vi "PostCopyScripting.vi"(10 "MetaDataObj":refnum<class "MetaDataObj.lvclass">, 11 "User Project":refnum<vi>) -> ()   [LabVIEW 2019, in "MetaDataObj.Instrument.lvclass"]
uses:
  MetaDataObj.Instrument.lvclass
  <resource>/dialog/NewProjectWizard/MetaDataObj/MetaDataObj.lvclass
  <userlib>/_MGI/File/MGI Create Directory Chain Behavior Enum.ctl
panel:
  out "Status":string
  # "Creating Project..."
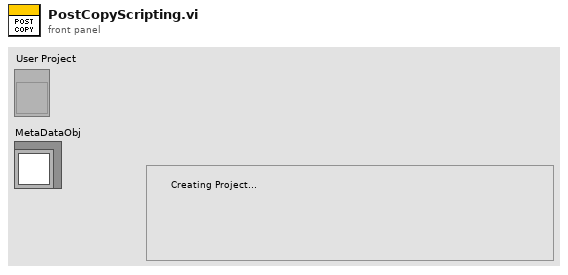
[diagram p1: front panel]
types:
  T1 = enum32{"Invalid", "Standard", "Closed", "Hidden", "Minimized", "Maximized"}
  T2 = enum32{"invalid app kind", "Development System", "Run Time System", "Student Edition", "Embedded LabVIEW", "Evaluation", "Custom"}
  T3 = typedef "MGI Create Directory Chain Behavior Enum.ctl" = enum16{"Auto Detect", "Path Contains a File", "Path Does Not Contain a File"}
  T4 = cluster{"Core":cluster{"Current VI Reference":refnum<vi>, "Close Panel on Exit?":bool}, "ProjectTemplate":path, "New Project Folder":path, "New Project File":path}
  T5 = cluster{"Current VI Reference":refnum<vi>, "Close Panel on Exit?":bool}
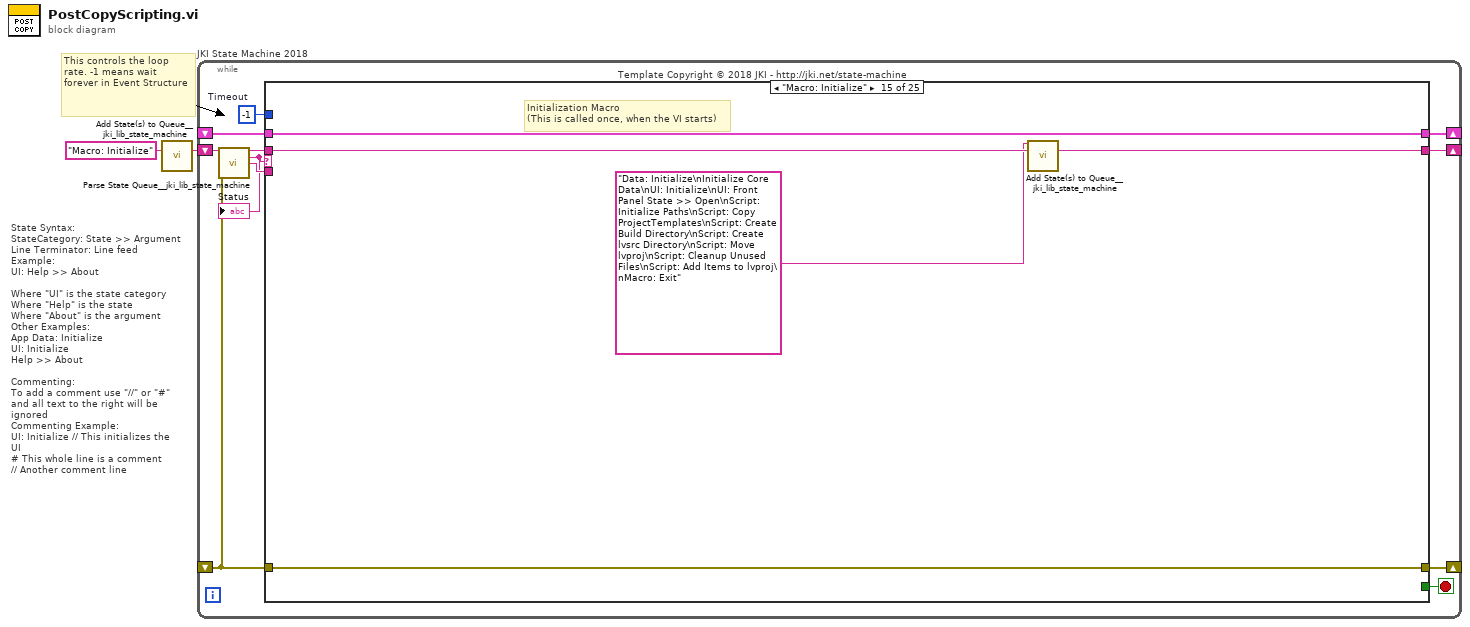
[diagram p0: block diagram]
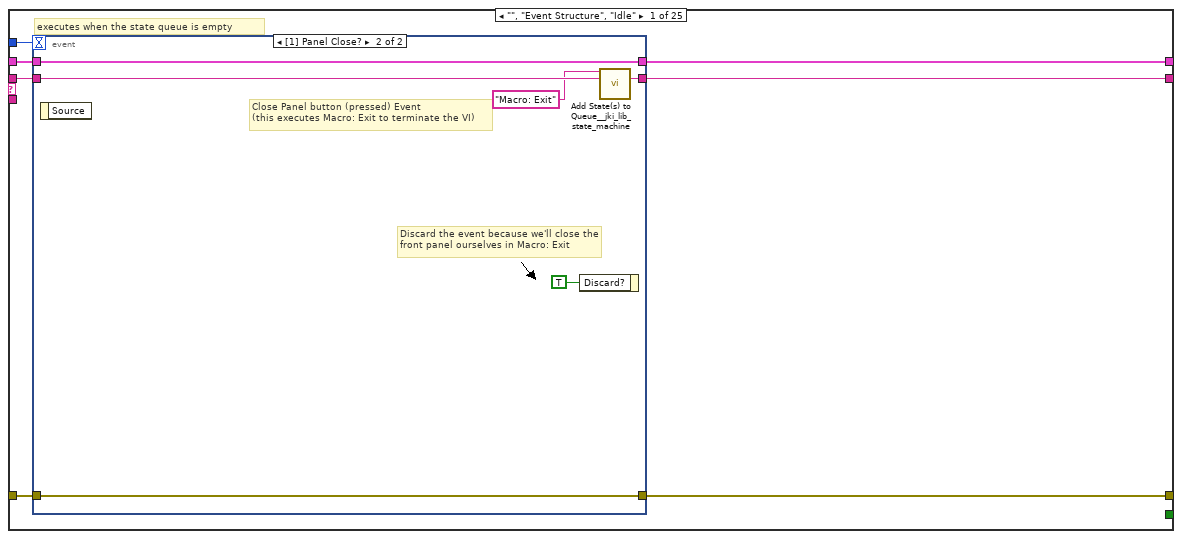
[diagram p2: hidden frame]
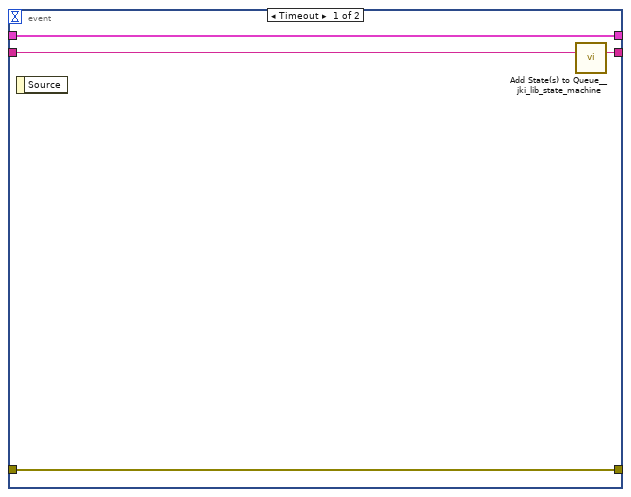
[diagram p3: hidden frame]
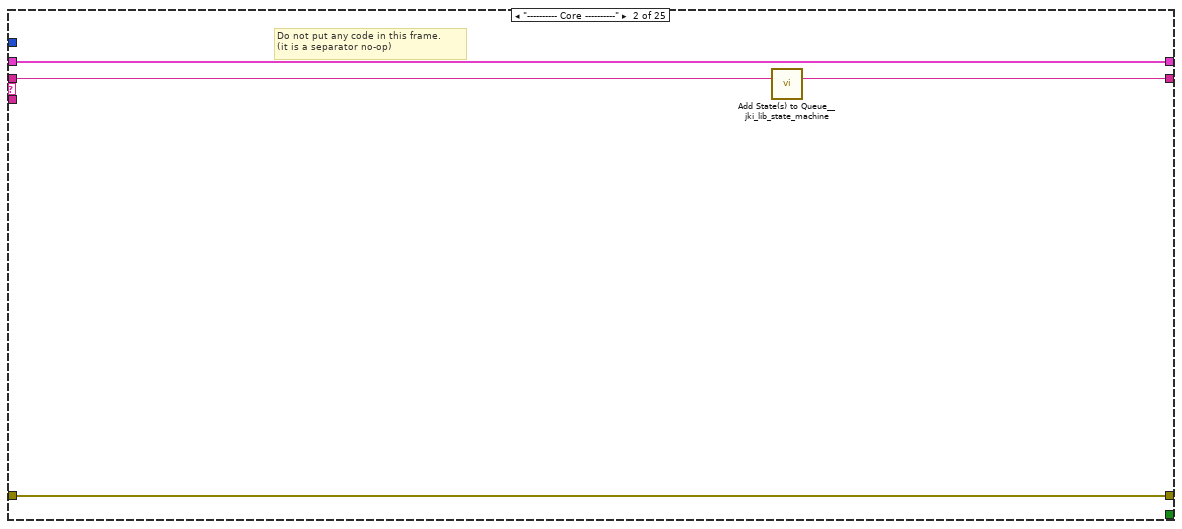
[diagram p4: hidden frame]
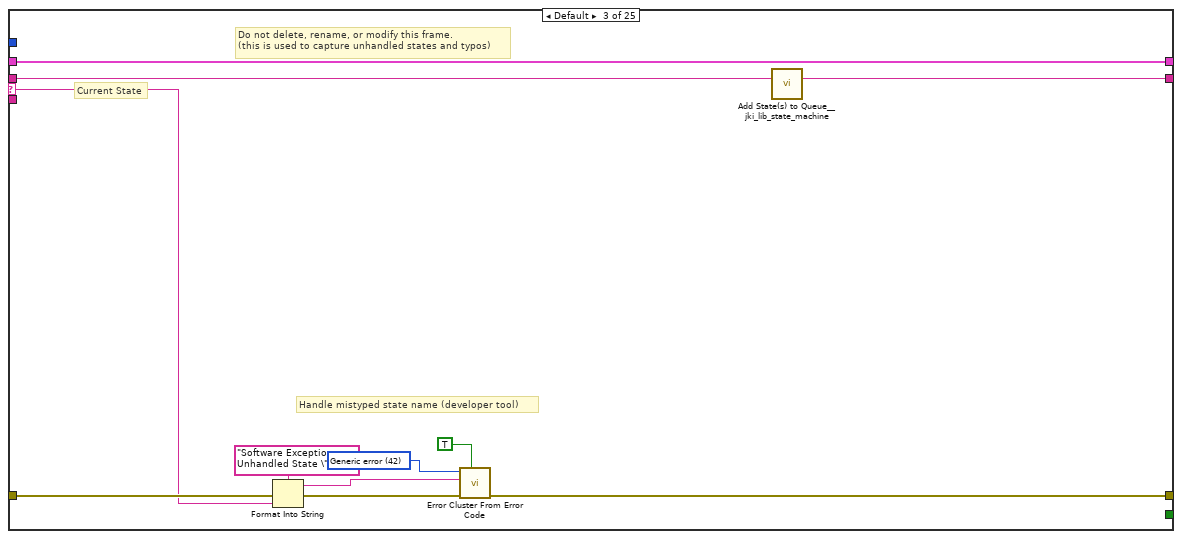
[diagram p5: hidden frame]
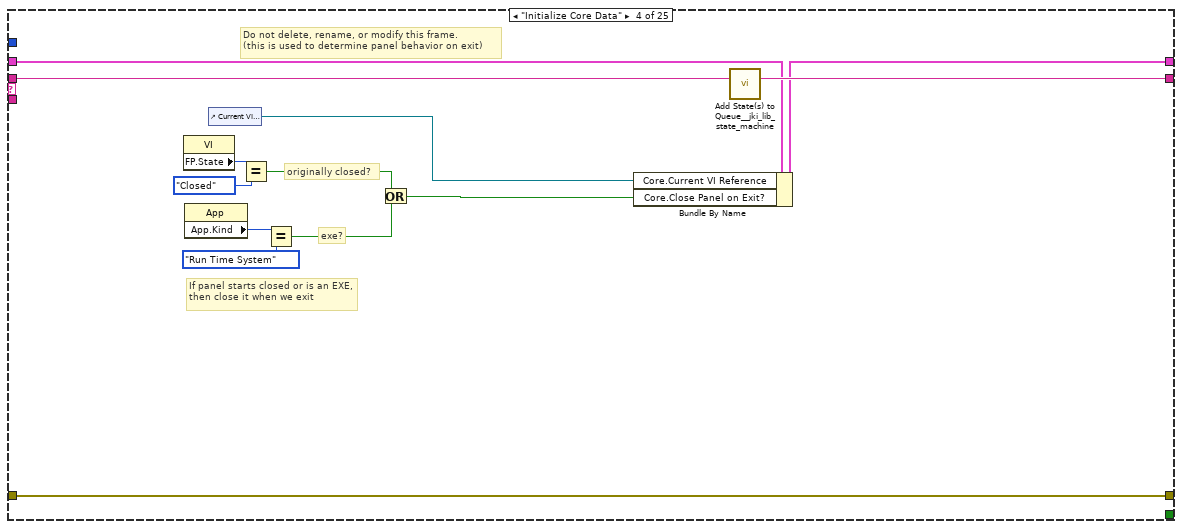
[diagram p6: hidden frame]
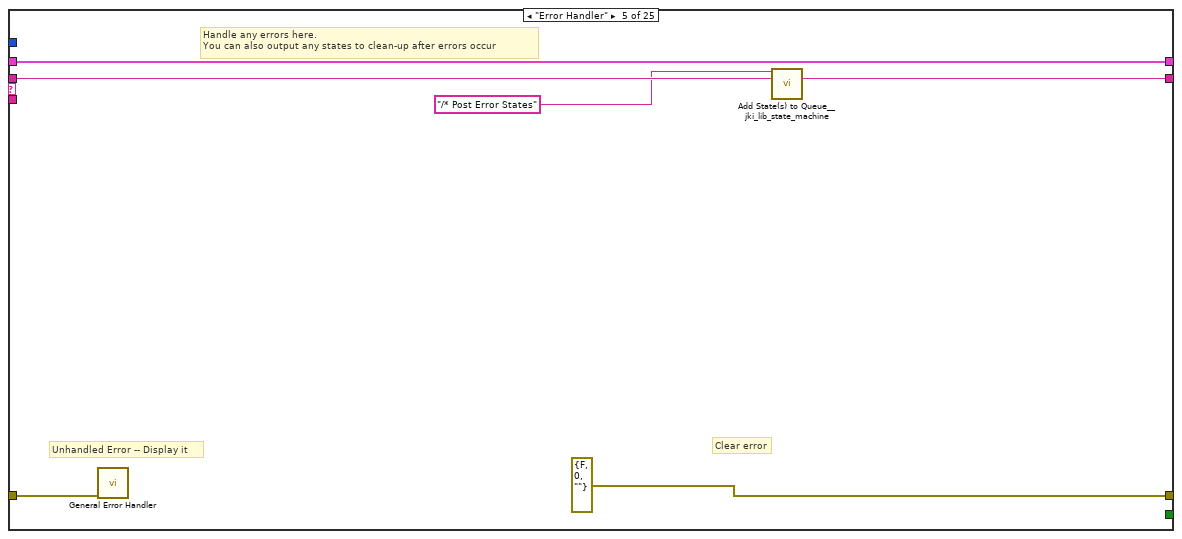
[diagram p7: hidden frame]
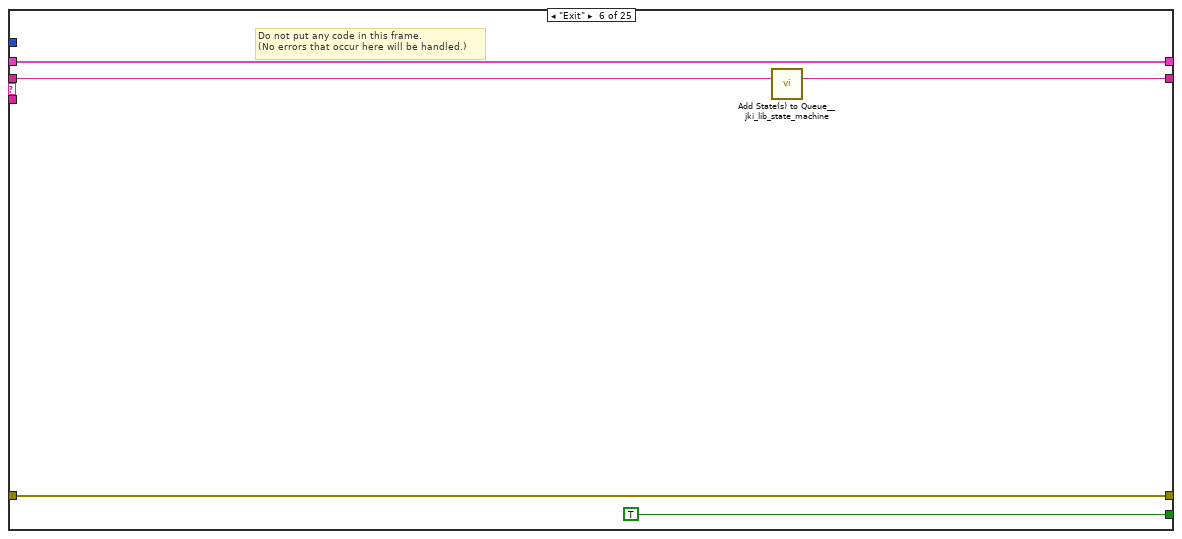
[diagram p8: hidden frame]
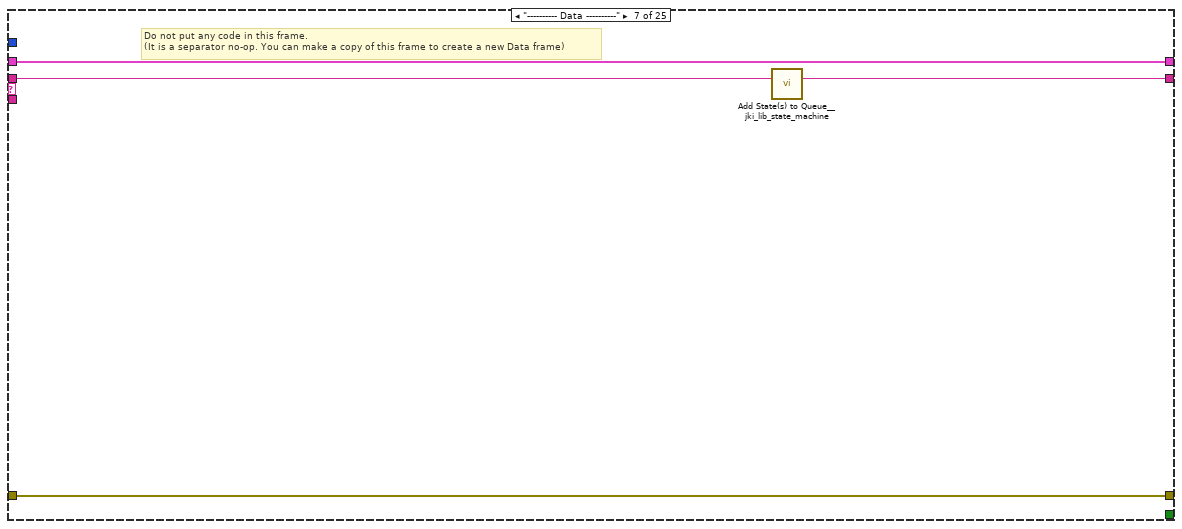
[diagram p9: hidden frame]
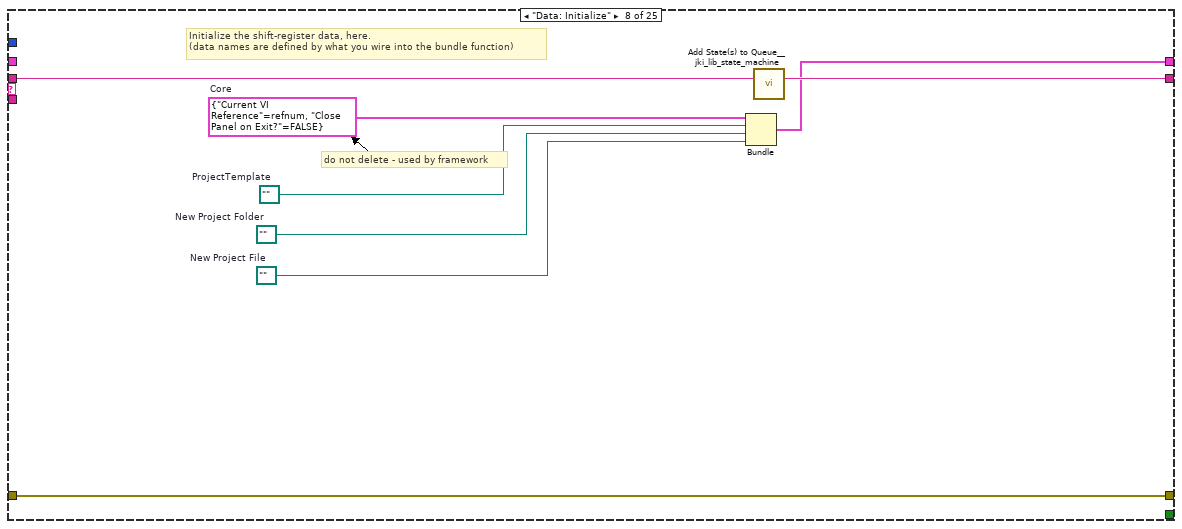
[diagram p10: hidden frame]
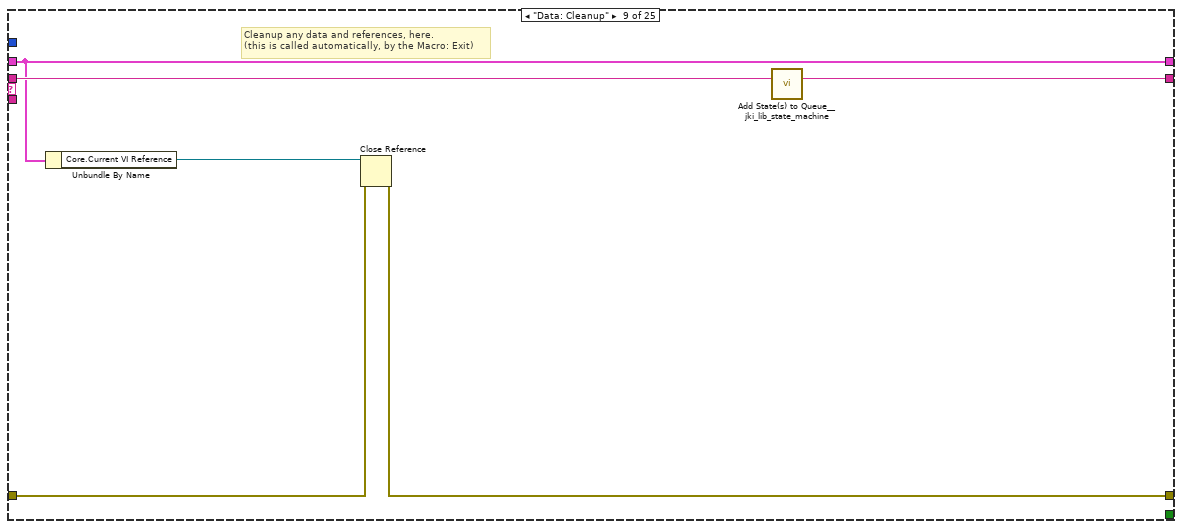
[diagram p11: hidden frame]
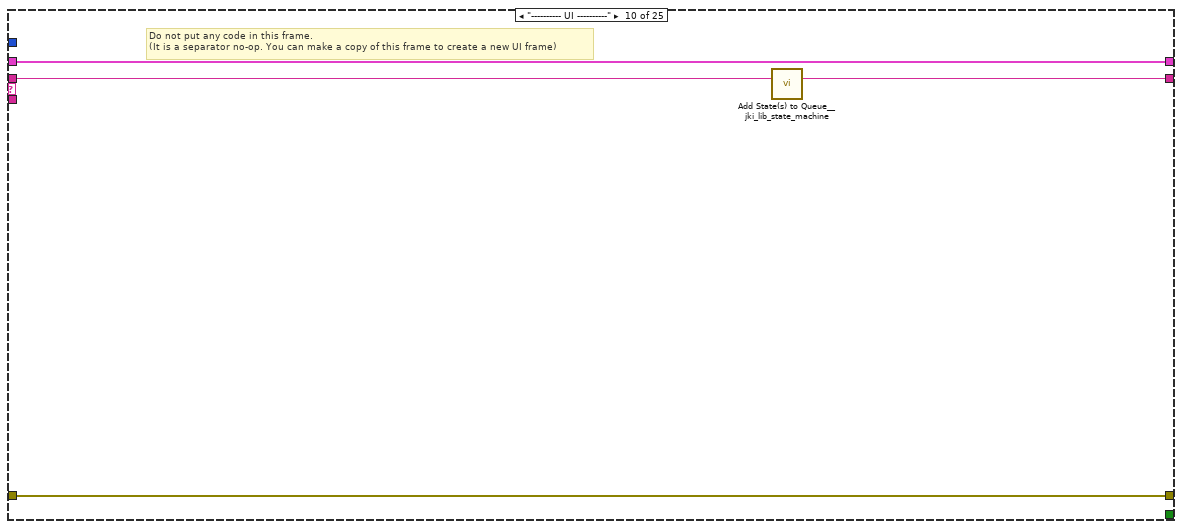
[diagram p12: hidden frame]
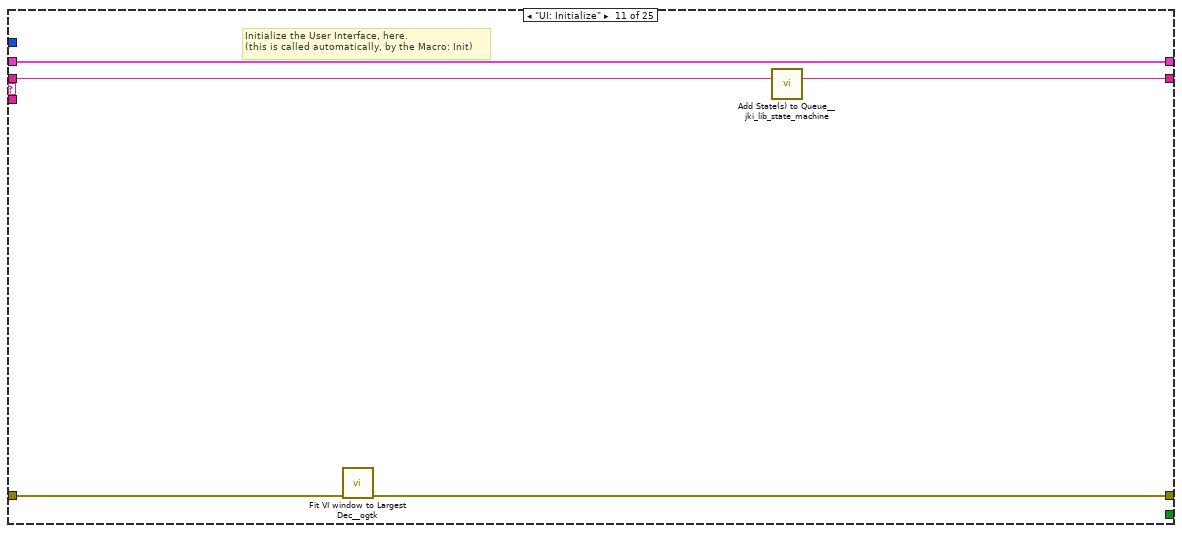
[diagram p13: hidden frame]
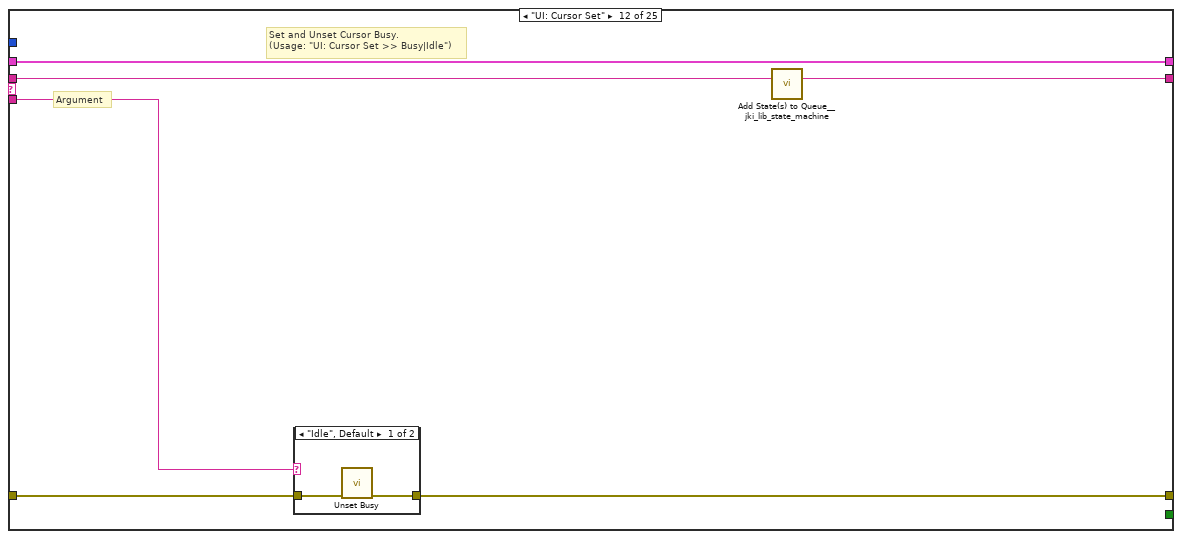
[diagram p14: hidden frame]
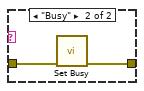
[diagram p15: hidden frame]
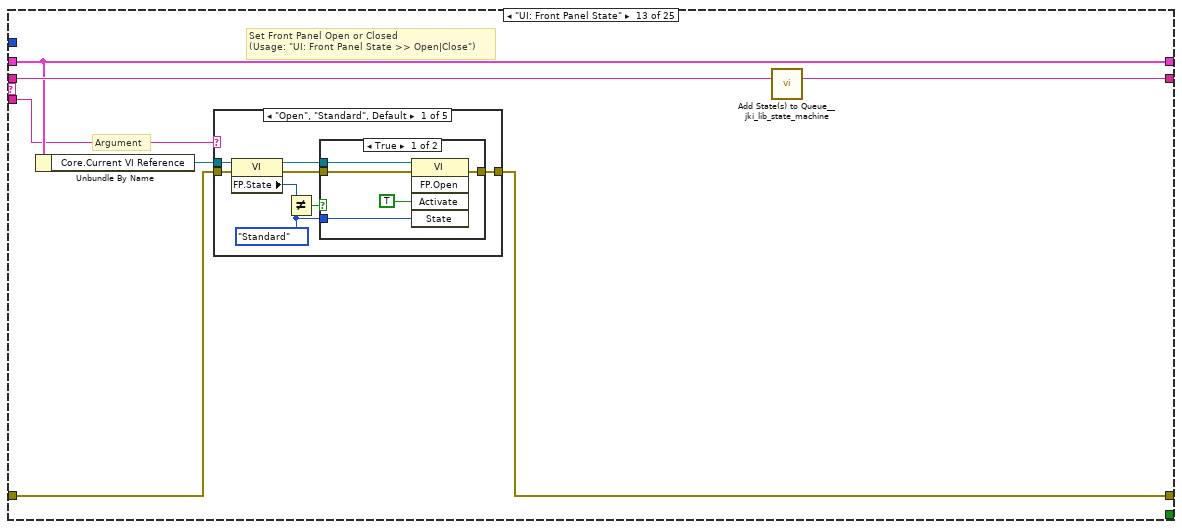
[diagram p16: hidden frame]
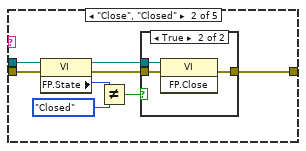
[diagram p18: hidden frame]
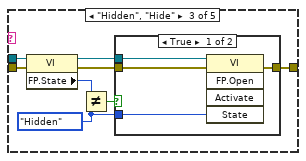
[diagram p20: hidden frame]
diagram:
  # "State Syntax:\nStateCategory: State >> Argument\nLine Terminator: Line feed\nExample:\nUI: Help >> About\n\nWhere \"UI\" is the state category\nWhere \"Help\" is the state\nWhere \"About\" is the argument\nOther Examples:\nApp Data: Initialize\nUI: Initialize\nHelp >> About\n\nCommenting:\nTo add a comment use \"//\" or \"#\" and all text to the right will be ignored\nCommenting Example:\nUI: Initialize // This initializes the UI\n# This whole line is a comment\n// Another comment line"
  # "This controls the loop rate. -1 means wait forever in Event Structure"
  n1 = call <vilib>:"Add State(s) to Queue__jki_lib_state_machine.vi"("State(s) in (\"\")"="Macro: Initialize") -> ("States Out"=w1:string)  [unwired: 14 in]
  n2 = while "JKI State Machine 2018" {
    shift-right: [w7] -> _
    shift-left: _ -> [w6]
    shift-right: [w10] -> _
    shift-left: _ -> [w4]
    shift-right: [w9] -> _
    shift-left: w1 -> [w11]
    stop <- w8 stop-if-true
    w5 = -1  # Timeout
    # "Template Copyright © 2018 JKI - http://jki.net/state-machine"
    n3 = call <vilib>:"Parse State Queue__jki_lib_state_machine.vi"("State Queue"=w11, "Error In (no error)"=w4) -> ("Remaining States"=w13:string, "Current State"=w3:string, "Arguments"=w12:string)  [unwired: 11 in]
    "Status" <- w3
    n4 = case shown="\"Macro: Initialize\"" w3 {
      selector: w3 -> [_ _ w35 _ _ _ _ _ _ _ _ _ _ _ _ _ _ _ _ _ _ _ _ _ _]
      tunnel: w13 -> [w20 w34 w39 w58 w64 w69 w73 w81 w87 w91 w96 w102 w113 w182 w187 w197 w201 w208 w223 w231 w269 w284 w300 w310 w338]
      tunnel: w12 -> [_ _ _ _ _ _ _ _ _ _ _ w97 w108 _ _ _ _ _ _ _ _ _ _ _ _]
      tunnel: w6 -> [w18 w31 w37 w51 w61 w67 w70 _ w82 w88 w94 w100 w110 w179 w184 w194 w198 w203 w217 w227 w263 w280 w287 w308 w336]
      tunnel: [w17 w32 w41 w55 errorcluster {"status"=FALSE, "code"=0, "source"=""} ("error out") w66 w71 w75 w83 w89 w92 w98 w107 w180 w185 w195 w199 w206 w221 w228 w261 w278 w289 w307 w320] -> w10
      tunnel: w4 -> [w16 w32 w40 w55 w60 w66 w71 w75 w84 w89 w93 w99 w111 w180 w185 w195 w199 w206 w221 w229 w262 w279 w290 w306 w335]
      tunnel: [w19 w33 w38 w57 w63 w68 w72 w80 w86 w90 w95 w101 w112 w181 w186 w196 w200 w207 w222 w230 w268 w283 w299 w309 w337] -> w9
      tunnel: [_ _ _ _ _ TRUE _ _ _ _ _ _ _ _ _ _ _ _ _ _ _ _ _ _ _] -> w8
      tunnel: [w15 w31 w37 w56 w61 w67 w70 w79 w82 w88 w94 w100 w110 w179 w184 w194 w198 w202 w216 w227 w263 w280 w286 w308 w336] -> w7
      tunnel: w5 -> [w14 _ _ _ _ _ _ _ _ _ _ _ _ _ _ _ _ _ _ _ _ _ _ _ _]
      frame "", "Event Structure", "Idle" {
        # "executes when the state queue is empty"
        n5 = event shown="[1] Panel Close?" {
          selector: _ -> [_ _]
          dyn-events: _ -> [_ _]
          timeout: w14 -> [_ _]
          tunnel: w20 -> [w24 w30]
          tunnel: [w23 w29] -> w19
          tunnel: w18 -> [w21 w27]
          tunnel: [w22 w28] -> w17
          tunnel: w16 -> [w22 w28]
          tunnel: [w21 w27] -> w15
          event Timeout {
            n6 = event-data() -> ()  [unwired: 1 in, 1 out]
            n7 = call <vilib>:"Add State(s) to Queue__jki_lib_state_machine.vi"("State(s) in (\"\")"=w24) -> ("States Out"=w23:string)  [unwired: 14 in]
          }
          event Panel Close? {
            # "Discard the event because we'll close the front panel ourselves in Macro: Exit"
            # "Close Panel button (pressed) Event\n(this executes Macro: Exit to terminate the VI)"
            n8 = event-data() -> ()  [unwired: 1 in, 1 out]
            n9 = event-data("Discard?"=TRUE) -> ()  [unwired: 1 in, 1 out]
            n10 = call <vilib>:"Add State(s) to Queue__jki_lib_state_machine.vi"("State(s) in Front (\"\")"="Macro: Exit", "State(s) in (\"\")"=w30) -> ("States Out"=w29:string)  [unwired: 13 in]
          }
        }
      }
      frame "---------- Core ----------" {
        # "Do not put any code in this frame.\n(it is a separator no-op)"
        n11 = call <vilib>:"Add State(s) to Queue__jki_lib_state_machine.vi"("State(s) in (\"\")"=w34) -> ("States Out"=w33:string)  [unwired: 14 in]
      }
      frame Default {
        w44 = 42 items=["No error", "Argument error", "Memory is full", "Out of zone", "End of file", "File already open", "Generic file I/O error", "File not found", "File permission error", "Disk is full", "Duplicate path", "Too many files open", "System feature not enabled", "Resource file not found", "Cannot add resource", "Resource not found", "Image not found", "Image memory error", "Pen does not exist", "Config type invalid", "Config token not found", "Config parse error", "Config memory error", "Bad external code format", "Bad external code offset", "External code not present", "Null window", "Destroy window error", "Null menu", "Print aborted", "Bad print record", "Print driver error", "Windows error during printing", "Memory error during printing", "Print dialog error", "Generic print error", "Invalid device refnum", "Device not found", "Device parameter error", "Device unit error", "Cannot open device", "Device call aborted", "Generic error", "Cancelled by user", "Object ID too low", "Object ID too high", "Object not in heap", "Unknown heap", "Unknown object (invalid DefProc)", "Unknown object (DefProc not in table)", "Message out of range", "Invalid (null) method", "Unknown message", "Manager call not supported", "Bad address", "Network operation in progress", "Network operation timed out", "Connection is busy", "Network attribute not supported", "Network error", "Address in use", "System out of memory", "Connection aborted", "Connection refused", "Not connected", "Already connected", "Connection closed", "Initialization error (interapplication manager)", "Bad occurrence", "Wait on unbound occurrence handler", "Occurrence queue overflow", "Datalog type conflict", "Unused", "Unrecognized type (interapplication manager)", "Memory corrupt", "Failed to make temporary DLL", "Old CIN version", "Drag socket not found", "Failed to load drop-object", "Failed to register OLE object", "Failed to release OLE object", "Format specifier type mismatch", "Unknown format specifier", "Too few format specifiers", "Too many format specifiers", "Scan failed", "Newer CIN version", "Error converting to variant", "Runtime menu error", "Password tampered", "Variant attribute not found", "Incompatible variant data type", "Event data is not available", "Event Store is not present", "Occurrence is not found", "Event Queue is not created", "Event info is not available", "Refnum passed is NULL", "Error retrieving Class GUID", "Error retrieving CoClass GUID", "Error retrieving TypeLib GUID.", "Bad built application magic bytes.", "Specific driver is different from the specific driver associated with the Logical Name.", "There is no session opened to the class driver.", "Max Error", "MAX - Error with config objects", "MAX - Error loading configuration", "MAX - Group not supported"]
        # "Current State"
        # "Do not delete, rename, or modify this frame.\n(this is used to capture unhandled states and typos)"
        # "Handle mistyped state name (developer tool)"
        n12 = Format Into String(format string="Software Exception: Unhandled State \"%s\"." ("message"), error in=w40, w35) -> (resulting string=w43:string, error out=w42:errorcluster)  [unwired: 1 in]
        n13 = call <vilib>:"Error Cluster From Error Code.vi"("show call chain? (False)"=TRUE, "error in (no error)"=w42, "error message (\"\")"=w43, "error code (0)"=w44) -> ("error out"=w41:errorcluster)  [unwired: 5 in]
        n14 = call <vilib>:"Add State(s) to Queue__jki_lib_state_machine.vi"("State(s) in (\"\")"=w39) -> ("States Out"=w38:string)  [unwired: 14 in]
      }
      frame "Initialize Core Data" {
        # "Do not delete, rename, or modify this frame.\n(this is used to determine panel behavior on exit)"
        # "originally closed?"
        # "exe?"
        # "If panel starts closed or is an EXE, then close it when we exit"
        n15 = property class="VI"() -> ("FP.State"=w48:T1)  [unwired: 2 in, 2 out]
        n16 = property class="App"() -> ("App.Kind"=w54:T2)  [unwired: 2 in, 2 out]
        n17 = control-ref of="Current VI Reference"() -> (w49:refnum<vi>)
        n18 = Equal?(x=w48, y=T1."Closed" ("Front Panel Window:State")) -> (x = y?=w46:bool)
        n19 = Equal?(x=w54, y=T2."Run Time System" ("Application:Kind")) -> (x = y?=w52:bool)
        n20 = Or(x=w46, y=w52) -> (x .or. y?=w50:bool)
        n21 = Bundle By Name(cluster=w51, "Core.Current VI Reference"=w49, "Core.Close Panel on Exit?"=w50) -> (w56:T4)
        n22 = call <vilib>:"Add State(s) to Queue__jki_lib_state_machine.vi"("State(s) in (\"\")"=w58) -> ("States Out"=w57:string)  [unwired: 14 in]
      }
      frame "Error Handler" {
        # "Unhandled Error -- Display it"
        # "Handle any errors here.\nYou can also output any states to clean-up after errors occur"
        # "Clear error"
        n23 = call <vilib>:"General Error Handler.vi"("error in (no error)"=w60) -> ()  [unwired: 10 in, 5 out]
        n24 = call <vilib>:"Add State(s) to Queue__jki_lib_state_machine.vi"("State(s) in Front (\"\")"="/* Post Error States", "State(s) in (\"\")"=w64) -> ("States Out"=w63:string)  [unwired: 13 in]
      }
      frame "Exit" {
        # "Do not put any code in this frame.\n(No errors that occur here will be handled.)"
        n25 = call <vilib>:"Add State(s) to Queue__jki_lib_state_machine.vi"("State(s) in (\"\")"=w69) -> ("States Out"=w68:string)  [unwired: 14 in]
      }
      frame "---------- Data ----------" {
        # "Do not put any code in this frame.\n(It is a separator no-op. You can make a copy of this frame to create a new Data frame)"
        n26 = call <vilib>:"Add State(s) to Queue__jki_lib_state_machine.vi"("State(s) in (\"\")"=w73) -> ("States Out"=w72:string)  [unwired: 14 in]
      }
      frame "Data: Initialize" {
        w74 = path ""  # New Project File
        w76 = path ""  # ProjectTemplate
        w77 = path ""  # New Project Folder
        w78 = T5 {"Current VI Reference"=refnum, "Close Panel on Exit?"=FALSE}  # Core
        # "do not delete - used by framework"
        # "Initialize the shift-register data, here.\n(data names are defined by what you wire into the bundle function)"
        n27 = Bundle("Core"=w78, "ProjectTemplate"=w76, "New Project Folder"=w77, "New Project File"=w74) -> (w79:T4)  [unwired: 1 in]
        n28 = call <vilib>:"Add State(s) to Queue__jki_lib_state_machine.vi"("State(s) in (\"\")"=w81) -> ("States Out"=w80:string)  [unwired: 14 in]
      }
      frame "Data: Cleanup" {
        # "Cleanup any data and references, here.\n(this is called automatically, by the Macro: Exit)"
        n29 = Unbundle By Name(w82) -> ("Core.Current VI Reference"=w85:refnum<vi>)
        n30 = Close Reference(reference=w85, error in (no error)=w84) -> (error out=w83:errorcluster)
        n31 = call <vilib>:"Add State(s) to Queue__jki_lib_state_machine.vi"("State(s) in (\"\")"=w87) -> ("States Out"=w86:string)  [unwired: 14 in]
      }
      frame "---------- UI ----------" {
        # "Do not put any code in this frame.\n(It is a separator no-op. You can make a copy of this frame to create a new UI frame)"
        n32 = call <vilib>:"Add State(s) to Queue__jki_lib_state_machine.vi"("State(s) in (\"\")"=w91) -> ("States Out"=w90:string)  [unwired: 14 in]
      }
      frame "UI: Initialize" {
        # "Initialize the User Interface, here.\n(this is called automatically, by the Macro: Init)"
        n33 = call <userlib>:"Fit VI window to Largest Dec__ogtk.vi"("error in (no error)"=w93) -> ("error out"=w92:errorcluster)  [unwired: 5 in, 1 out]
        n34 = call <vilib>:"Add State(s) to Queue__jki_lib_state_machine.vi"("State(s) in (\"\")"=w96) -> ("States Out"=w95:string)  [unwired: 14 in]
      }
      frame "UI: Cursor Set" {
        # "Argument"
        # "Set and Unset Cursor Busy.\n(Usage: \"UI: Cursor Set >> Busy|Idle\")"
        n35 = case shown="\"Idle\", Default" w97 {
          tunnel: w99 -> [w104 w106]
          tunnel: [w103 w105] -> w98
          frame "Idle", Default {
            n36 = call <vilib>:"Unset Busy.vi"("error in (no error)"=w104) -> ("error out"=w103:errorcluster)  [unwired: 10 in]
          }
          frame "Busy" {
            n37 = call <vilib>:"Set Busy.vi"("error in (no error)"=w106) -> ("error out"=w105:errorcluster)  [unwired: 9 in, 1 out]
          }
        }
        n38 = call <vilib>:"Add State(s) to Queue__jki_lib_state_machine.vi"("State(s) in (\"\")"=w102) -> ("States Out"=w101:string)  [unwired: 14 in]
      }
      frame "UI: Front Panel State" {
        # "Argument"
        # "Set Front Panel Open or Closed\n(Usage: \"UI: Front Panel State >> Open|Close\")"
        n39 = Unbundle By Name(w110) -> ("Core.Current VI Reference"=w109:refnum<vi>)
        n40 = case shown="\"Open\", \"Standard\", Default" w108 {
          tunnel: w111 -> [w119 w134 w145 w158 w171]
          tunnel: [w121 w135 w147 w160 w173] -> w107
          tunnel: w109 -> [w120 w132 w146 w159 w172]
          frame "Open", "Standard", Default {
            w114 = T1."Standard" ("State")
            n41 = property class="VI"(reference=w120, error in=w119) -> (reference out=w117:refnum<vi>, error out=w118:errorcluster, "FP.State"=w116:T1)
            n42 = Not Equal?(x=w116, y=w114) -> (x != y?=w115:bool)
            n43 = case shown="True" w115 {
              tunnel: [w125 w127] -> w121
              tunnel: w118 -> [w124 w127]
              tunnel: w117 -> [w123 _]
              tunnel: w114 -> [w122 _]
              frame True {
                n44 = invoke class="VI" method="FP.Open"(reference=w123, error in=w124, "Activate"=TRUE, "State"=w122) -> (error out=w125:errorcluster)  [unwired: 1 in, 4 out]
              }
              frame False {
              }
            }
          }
          frame "Close", "Closed" {
            n45 = property class="VI"(reference=w132, error in=w134) -> (reference out=w131:refnum<vi>, error out=w133:errorcluster, "FP.State"=w129:T1)
            n46 = Not Equal?(x=w129, y=T1."Closed" ("Front Panel Window:State")) -> (x != y?=w128:bool)
            n47 = case shown="True" w128 {
              tunnel: [w136 w139] -> w135
              tunnel: w133 -> [w136 w138]
              tunnel: w131 -> [_ w137]
              frame False {
              }
              frame True {
                n48 = invoke class="VI" method="FP.Close"(reference=w137, error in=w138) -> (error out=w139:errorcluster)  [unwired: 1 in, 2 out]
              }
            }
          }
          frame "Hidden", "Hide" {
            w140 = T1."Hidden" ("State")
            n49 = property class="VI"(reference=w146, error in=w145) -> (reference out=w143:refnum<vi>, error out=w144:errorcluster, "FP.State"=w142:T1)
            n50 = Not Equal?(x=w142, y=w140) -> (x != y?=w141:bool)
            n51 = case shown="True" w141 {
              tunnel: [w151 w152] -> w147
              tunnel: w144 -> [w150 w152]
              tunnel: w143 -> [w149 _]
              tunnel: w140 -> [w148 _]
              frame True {
                n52 = invoke class="VI" method="FP.Open"(reference=w149, error in=w150, "State"=w148) -> (error out=w151:errorcluster)  [unwired: 2 in, 4 out]
              }
              frame False {
              }
            }
          }
          frame "Minimize", "Minimized" {
            w153 = T1."Minimized" ("State")
            n53 = property class="VI"(reference=w159, error in=w158) -> (reference out=w156:refnum<vi>, error out=w157:errorcluster, "FP.State"=w155:T1)
            n54 = Not Equal?(x=w155, y=w153) -> (x != y?=w154:bool)
            n55 = case shown="True" w154 {
              tunnel: [w164 w165] -> w160
              tunnel: w157 -> [w163 w165]
              tunnel: w156 -> [w162 _]
              tunnel: w153 -> [w161 _]
              frame True {
                n56 = invoke class="VI" method="FP.Open"(reference=w162, error in=w163, "State"=w161) -> (error out=w164:errorcluster)  [unwired: 2 in, 4 out]
              }
              frame False {
              }
            }
          }
          frame "Maximize", "Maximized" {
            w166 = T1."Maximized" ("State")
            n57 = property class="VI"(reference=w172, error in=w171) -> (reference out=w169:refnum<vi>, error out=w170:errorcluster, "FP.State"=w168:T1)
            n58 = Not Equal?(x=w168, y=w166) -> (x != y?=w167:bool)
            n59 = case shown="True" w167 {
              tunnel: [w177 w178] -> w173
              tunnel: w170 -> [w176 w178]
              tunnel: w169 -> [w175 _]
              tunnel: w166 -> [w174 _]
              frame True {
                n60 = invoke class="VI" method="FP.Open"(reference=w175, error in=w176, "State"=w174) -> (error out=w177:errorcluster)  [unwired: 2 in, 4 out]
              }
              frame False {
              }
            }
          }
        }
        n61 = call <vilib>:"Add State(s) to Queue__jki_lib_state_machine.vi"("State(s) in (\"\")"=w113) -> ("States Out"=w112:string)  [unwired: 14 in]
      }
      frame "---------- Macro ----------" {
        # "Do not put any code in this frame.\n(It is a separator no-op. You can make a copy of this frame to create a new Macro frame)"
        n62 = call <vilib>:"Add State(s) to Queue__jki_lib_state_machine.vi"("State(s) in (\"\")"=w182) -> ("States Out"=w181:string)  [unwired: 14 in]
      }
      frame "Macro: Initialize" {
        # "Initialization Macro\n(This is called once, when the VI starts)"
        n63 = call <vilib>:"Add State(s) to Queue__jki_lib_state_machine.vi"("State(s) in Front (\"\")"="Data: Initialize\nInitialize Core Data\nUI: Initialize\nUI: Front Panel State >> Open\nScript: Initialize Paths\nScript: Copy ProjectTemplates\nScript: Create Build Directory\nScript: Create lvsrc Directory\nScript: Move lvproj\nScript: Cleanup Unused Files\nScript: Add Items to lvproj\nMacro: Exit", "State(s) in (\"\")"=w187) -> ("States Out"=w186:string)  [unwired: 13 in]
      }
      frame "Macro: Exit" {
        # "Exit Macro\n(This is called once, when the VI exits)"
        n64 = Unbundle By Name(w194) -> ("Core.Close Panel on Exit?"=w193:bool)
        n65 = Select(t="UI: Front Panel State >> Close", s=w193, f="") -> (s? t:f=w190:string)
        n66 = call <vilib>:"Add State(s) to Queue__jki_lib_state_machine.vi"("State(s) in (\"\")"=w190, "State(s) at Back (\"\")"="Data: Cleanup\nExit") -> ("States Out"=w188:string)  [unwired: 13 in]
        n67 = call <vilib>:"Add State(s) to Queue__jki_lib_state_machine.vi"("State(s) in Front (\"\")"=w188, "State(s) in (\"\")"=w197) -> ("States Out"=w196:string)  [unwired: 13 in]
      }
      frame "---------- Script ----------" {
        # "Template Separator\n(You can make a copy of, or modify, this frame)"
        n68 = call <vilib>:"Add State(s) to Queue__jki_lib_state_machine.vi"("State(s) in (\"\")"=w201) -> ("States Out"=w200:string)  [unwired: 14 in]
      }
      frame "Script: Template" {
        # "Your code here.\n(You can make a copy of, or modify, this frame)"
        n69 = Unbundle By Name(w203) -> ("ProjectTemplate"=w205:path, "New Project Folder"=w204:path)
        n70 = Bundle By Name(cluster=w203, "ProjectTemplate"=w205, "New Project Folder"=w204) -> (w202:T4)
        n71 = call <vilib>:"Add State(s) to Queue__jki_lib_state_machine.vi"("State(s) in (\"\")"=w208) -> ("States Out"=w207:string)  [unwired: 14 in]
      }
      frame "Script: Initialize Paths" {
        w210 = refnum<class "MetaDataObj.Instrument.lvclass"> refnum  # MetaDataObj.Instrument.lvclass
        # "path to new project source"
        # "path to ProjectTemplate location"
        # "LabVIEW directory"
        # "Initialize Paths.\n(description)"
        n72 = property class="Project"(reference="User Project") -> (reference out=w214:refnum<vi>, error out=w213:errorcluster, "Path"=w209:path)  [unwired: 1 in]
        n73 = Default Directory() -> (w220:path)
        n74 = To More Specific Class(target class=w210, reference="MetaDataObj") -> ()  [unwired: 1 in, 2 out]
        n75 = Build Path(base path=w220, name or relative path="ProjectTemplates\\Source\\LevyLab\\Instrument\\project files") -> (appended path=w218:path)
        n76 = Close Reference(reference=w214, error in (no error)=w213) -> ()  [unwired: 1 out]
        n77 = Strip Path(path=w209) -> (stripped path=w215:path)  [unwired: 1 out]
        n78 = Bundle By Name(cluster=w217, "ProjectTemplate"=w218, "New Project Folder"=w215) -> (w216:T4)
        n79 = call <vilib>:"Add State(s) to Queue__jki_lib_state_machine.vi"("State(s) in (\"\")"=w223) -> ("States Out"=w222:string)  [unwired: 14 in]
      }
      frame "Script: Copy ProjectTemplates" {
        # "Copy code from ProjectTemplate to Source.\n(copy fiels that the Create Project dialog won't copy)"
        n80 = Unbundle By Name(w227) -> ("ProjectTemplate"=w225:path, "New Project Folder"=w226:path)
        n81 = for {
          tunnel: w226 -> [w242]
          shift-right: [w235] -> w228
          shift-left: w229 -> [w238]
          tunnel: string[] ["", "build support"] -> [w232] mode=indexing
          tunnel: w225 -> [w234]
          n82 = case shown="Default" w232 {
            selector: w232 -> [_ w246]
            tunnel: w234 -> [w245 w248]
            tunnel: [w245 w247] -> w233
            frame "" {
            }
            frame Default {
              n83 = Build Path(base path=w248, name or relative path=w246) -> (appended path=w247:path)
            }
          }
          n84 = case shown="Default" w232 {
            selector: w232 -> [_ w250]
            tunnel: w242 -> [w249 w252]
            tunnel: [w249 w251] -> w241
            frame "" {
            }
            frame Default {
              n85 = Build Path(base path=w252, name or relative path=w250) -> (appended path=w251:path)
            }
          }
          n86 = List Folder(path=w233, error in=w238) -> (path out=w244:path, filenames=w243:string[], error out=w237:errorcluster)  [unwired: 2 in, 1 out]
          n87 = call <userlib>:"MGI Create Directory Chain.vi"("Error In"=w237, "File Presence (Auto Detect)"=MGI_Create_Directory_Chain_Behavior_Enum."Auto Detect", "Path"=w241) -> ("Error Out"=w236:errorcluster, "Duplicate Path"=w240:path)  [unwired: 7 in]
          n88 = for {
            tunnel: w244 -> [w260]
            tunnel: w243 -> [w258] mode=indexing
            tunnel: w240 -> [w259]
            shift-right: [w253] -> w235
            shift-left: w236 -> [w256]
            n89 = Build Path(base path=w260, name or relative path=w258) -> (appended path=w254:path)
            n90 = Build Path(base path=w259, name or relative path=w258) -> (appended path=w255:path)
            n91 = Copy(8:w256, 9:TRUE ("overwrite (F)"), 10:w255, 11:w254) -> (0:w253:errorcluster)  [unwired: 1 in, 2 out]
          }
        }
        n92 = call <vilib>:"Add State(s) to Queue__jki_lib_state_machine.vi"("State(s) in (\"\")"=w231) -> ("States Out"=w230:string)  [unwired: 14 in]
      }
      frame "Script: Create Build Directory" {
        # "Create default builds/subfolder structure."
        n93 = Unbundle By Name(w263) -> ("New Project Folder"=w266:path)
        n94 = Build Path(base path=w266, name or relative path="builds") -> (appended path=w264:path)
        n95 = for {
          shift-right: [w270] -> w261
          shift-left: w262 -> [w274]
          tunnel: w264 -> [w273]
          tunnel: string[] ["7z Install", "Application", "Installer", "Latest", "Package"] -> [w272] mode=indexing
          tunnel: [w270] -> _ mode=indexing
          n96 = Build Path(base path=w273, name or relative path=w272) -> (appended path=w271:path)
          n97 = call <userlib>:"MGI Create Directory Chain.vi"("Error In"=w274, "File Presence (Auto Detect)"=MGI_Create_Directory_Chain_Behavior_Enum."Auto Detect", "Path"=w271) -> ("Error Out"=w270:errorcluster)  [unwired: 7 in, 1 out]
        }
        n98 = call <vilib>:"Add State(s) to Queue__jki_lib_state_machine.vi"("State(s) in (\"\")"=w269) -> ("States Out"=w268:string)  [unwired: 14 in]
      }
      frame "Script: Create lvsrc Directory" {
        # "Create lvsrc/ folder."
        n99 = Unbundle By Name(w280) -> ("New Project Folder"=w282:path)
        n100 = Build Path(base path=w282, name or relative path="lvsrc\\SMOs") -> (appended path=w276:path)
        n101 = call <userlib>:"MGI Create Directory Chain.vi"("Error In"=w279, "File Presence (Auto Detect)"=MGI_Create_Directory_Chain_Behavior_Enum."Auto Detect", "Path"=w276) -> ("Error Out"=w278:errorcluster)  [unwired: 7 in, 1 out]
        n102 = call <vilib>:"Add State(s) to Queue__jki_lib_state_machine.vi"("State(s) in (\"\")"=w284) -> ("States Out"=w283:string)  [unwired: 14 in]
      }
      frame "Script: Move lvproj" {
        # "Move *.lvproj from root to lvsrc/"
        n103 = Unbundle By Name(w287) -> ("New Project Folder"=w291:path)
        n104 = call <vilib>:"Recursive File List.vi"("pattern"="*.lvproj", "error in (no error)"=w290, "Folder Path"=w291) -> ("error out"=w294:errorcluster, "All Files in Dir"=w285:path[])  [unwired: 4 in, 3 out]
        n105 = Build Path(base path=w291, name or relative path="lvsrc") -> (appended path=w297:path)
        n106 = Index Array(array=w285) -> (element=w296:path)  [unwired: 1 in]
        n107 = Strip Path(path=w296) -> (name=w292:string)  [unwired: 1 out]
        n108 = Build Path(base path=w297, name or relative path=w292) -> (appended path=w298:path)
        n109 = Move(source path=w296, error in=w294, 10:w298) -> (error out=w289:errorcluster, 3:w288:path)  [unwired: 2 in, 1 out]
        n110 = Bundle By Name(cluster=w287, "New Project File"=w288) -> (w286:T4)
        n111 = call <vilib>:"Add State(s) to Queue__jki_lib_state_machine.vi"("State(s) in (\"\")"=w300) -> ("States Out"=w299:string)  [unwired: 14 in]
      }
      frame "Script: Cleanup Unused Files" {
        # "Delete uneeded files."
        n112 = Unbundle By Name(w308) -> ("New Project Folder"=w305:path)
        n113 = Build Array("*.aliases" ("pattern"), "*.lvlps" ("pattern"), "*.rename" ("pattern")) -> (w301:string[])
        n114 = for {
          tunnel: w305 -> [w312]
          shift-right: [w316] -> w307
          shift-left: w306 -> [w313]
          tunnel: w301 -> [w311] mode=indexing
          n115 = call <vilib>:"Recursive File List.vi"("pattern"=w311, "error in (no error)"=w313, "Folder Path"=w312) -> ("error out"=w315:errorcluster, "All Files in Dir"=w314:path[])  [unwired: 4 in, 3 out]
          n116 = for {
            tunnel: w314 -> [w319] mode=indexing
            shift-right: [w317] -> w316
            shift-left: w315 -> [w318]
            n117 = Delete(path (use dialog)=w319, error in=w318) -> (error out=w317:errorcluster)  [unwired: 3 in, 2 out]
          }
        }
        n118 = call <vilib>:"Add State(s) to Queue__jki_lib_state_machine.vi"("State(s) in (\"\")"=w310) -> ("States Out"=w309:string)  [unwired: 14 in]
      }
      frame "Script: Add Items to lvproj" {
        # "Add items to the Project"
        n119 = Unbundle By Name(w336) -> ("New Project Folder"=w332:path, "New Project File"=w330:path)
        n120 = invoke class="App" method="Project.Open"(error in=w335, "Path"=w330) -> (error out=w328:errorcluster, "Project:Open"=w329:refnum<vi>)  [unwired: 2 in, 2 out]
        n121 = invoke class="Project" method="Open Window"(reference=w329, error in=w328) -> (reference out=w327:refnum<vi>, error out=w326:errorcluster)  [unwired: 1 in, 1 out]
        n122 = property class="Project"(reference=w327, error in=w326) -> (reference out=w323:refnum<vi>, error out=w334:errorcluster, "My Computer"=w333:refnum<vi>)
        n123 = for "Add Folders" {
          tunnel: w334 -> [w349]
          tunnel: w333 -> [w347]
          tunnel: string[] ["build support", "lvsrc"] -> [w342] mode=indexing
          tunnel: w332 -> [w340]
          tunnel: [w344] -> w331
          n124 = Build Path(base path=w340, name or relative path=w342) -> (appended path=w339:path)
          n125 = invoke class="TargetItem" method="AddItem"(reference=w347, error in=w349, "Name"=w342, "Path"=w339, "Type"="Folder") -> (error out=w346:errorcluster, "AddItem"=w343:refnum<vi>)  [unwired: 1 in, 4 out]
          n126 = case shown="Default" w342 {
            tunnel: w346 -> [w351 w356]
            tunnel: [w351 w355] -> w345
            tunnel: w339 -> [_ w354]
            tunnel: w343 -> [w350 w353]
            tunnel: [w350 w352] -> w341
            frame "lvsrc" {
            }
            frame Default {
              n127 = call <vilib>:"Recursive File List.vi"("error in (no error)"=w356, "Folder Path"=w354) -> ("error out"=w358:errorcluster, "All Files in Dir"=w357:path[])  [unwired: 5 in, 3 out]
              n128 = for "Add Folder Contents" {
                tunnel: w353 -> [w360]
                tunnel: w357 -> [w363] mode=indexing
                tunnel: w358 -> [w365]
                tunnel: [w362] -> w355
                tunnel: [w359] -> w352
                n129 = invoke class="ProjectItem" method="AddFile"(reference=w360, error in=w365, "Path"=w363) -> (reference out=w359:refnum<vi>, error out=w364:errorcluster, "AddFile"=w361:refnum<vi>)  [unwired: 1 in, 1 out]
                n130 = Close Reference(reference=w361, error in (no error)=w364) -> (error out=w362:errorcluster)
              }
            }
          }
          n131 = Close Reference(reference=w341, error in (no error)=w345) -> (error out=w344:errorcluster)
        }
        n132 = Close Reference(reference=w333, error in (no error)=w331) -> (error out=w324:errorcluster)
        n133 = invoke class="Project" method="Save"(reference=w323, error in=w324) -> (reference out=w322:refnum<vi>, error out=w321:errorcluster)  [unwired: 2 in, 2 out]
        n134 = Close Reference(reference=w322, error in (no error)=w321) -> (error out=w320:errorcluster)
        n135 = call <vilib>:"Add State(s) to Queue__jki_lib_state_machine.vi"("State(s) in (\"\")"=w338) -> ("States Out"=w337:string)  [unwired: 14 in]
      }
    }
  }
